vi "Create Logger.vi"(8 "error in (no error)":errorcluster, 11 "Logger.Error in":refnum<class "Logger.Error.lvclass">) -> (0 "error out":errorcluster, 3 "Logger.Error out":refnum<class "Logger.Error.lvclass">)   [LabVIEW 2019, in "Logger.Error.lvlib" / "Logger.Error.lvclass"]
uses:
  Logger.Error.lvclass
  <vilib>/Utility/file.llb/Write Delimited Spreadsheet (string).vi
  <userlib>/LevyLab/Logger/Logger/Logger.lvclass
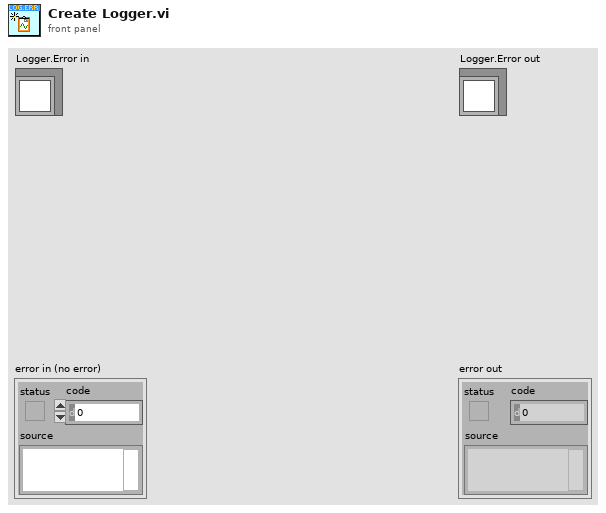
[diagram p1: front panel]
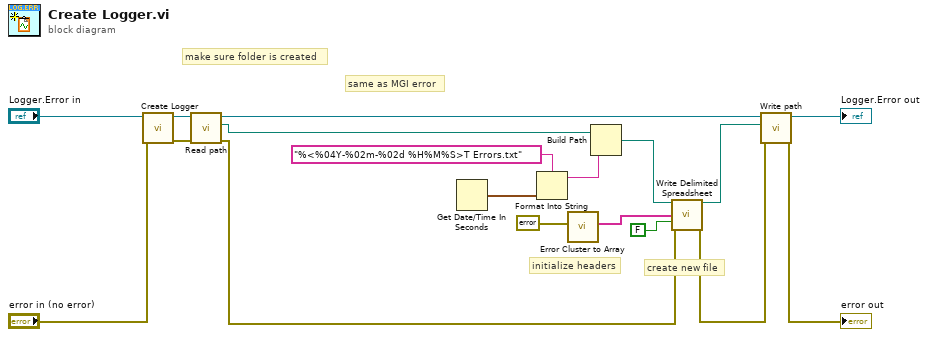
[diagram p0: block diagram]
diagram:
  # "make sure folder is created"
  # "same as MGI error"
  # "create new file"
  # "initialize headers"
  n1 = call-parent "Create Logger.vi"("error in (no error)"="error in (no error)", "Logger in"="Logger.Error in") -> ("error out"=w17:errorcluster, "Logger out"=w16:refnum<class "Logger.Error.lvclass">)  [unwired: 8 in]
  n2 = call-dynamic "Read path.vi"("error in (no error)"=w17, "Logger in"=w16) -> ("error out"=w1:errorcluster, "path"=w3:path, "Logger out"=w14:refnum<class "Logger.Error.lvclass">)  [unwired: 7 in]
  n3 = Get Date/Time In Seconds() -> (seconds since 1Jan1904=w11:timestamp)
  n4 = Format Into String(format string="%<%04Y-%02m-%02d %H%M%S>T Errors.txt", w11) -> (resulting string=w10:string)  [unwired: 2 in, 1 out]
  n5 = call "Error Cluster to Array.vi"("error in (no error)"=errorcluster {"status"=FALSE, "code"=0, "source"=""}) -> ("Error Array"=w6:string[])  [unwired: 10 in]
  n6 = Build Path(base path=w3, name or relative path=w10) -> (appended path=w8:path)
  n7 = call-poly <vilib>:"Write Delimited Spreadsheet.vi"("file path (dialog if empty)"=w8, "1D data"=w6, "append to file? (new file:F)"=FALSE, "error in (no error)"=w1) -> ("new file path (Not A Path if cancelled)"=w5:path, "error out"=w4:errorcluster)  [unwired: 10 in]
  n8 = call-dynamic "Write path.vi"("error in (no error)"=w4, "folder"=w5, "Logger in"=w14) -> ("error out"=→"error out":errorcluster, "Logger out"=→"Logger.Error out":refnum<class "Logger.Error.lvclass">)  [unwired: 7 in]
